vi "Check RPM.vi"(10 "Motor Input":dbl, 11 "RPM":dbl) -> (3 "RPM Drop":bool)   [LabVIEW 2013]
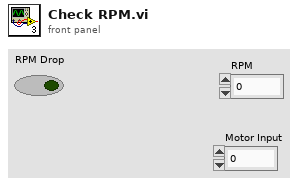
[diagram p1: front panel]
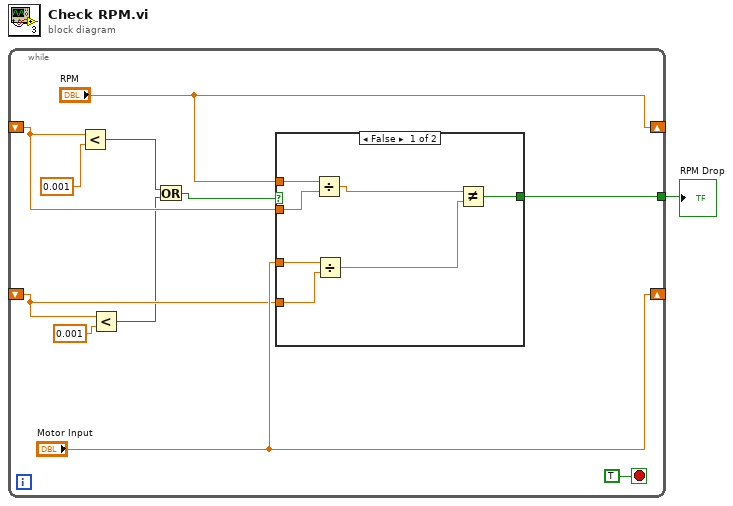
[diagram p0: block diagram]
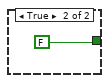
[diagram p2: hidden frame]
diagram:
  n1 = while {
    shift-right: ["RPM"] -> _
    shift-left: _ -> [w5]
    shift-right: ["Motor Input"] -> _
    shift-left: _ -> [w7]
    tunnel: [w9] -> w1
    stop <- TRUE stop-if-true
    n2 = Less?(x=w5, y=0.001) -> (x < y?=w4:bool)
    n3 = Less?(x=w7, y=0.001) -> (x < y?=w3:bool)
    n4 = Or(x=w4, y=w3) -> (x .or. y?=w2:bool)
    n5 = case shown="False" w2 {
      tunnel: [w19 FALSE] -> w9
      tunnel: "Motor Input" -> [w18 _]
      tunnel: w7 -> [w17 _]
      tunnel: "RPM" -> [w16 _]
      tunnel: w5 -> [w15 _]
      frame False {
        n6 = Divide(x=w16, y=w15) -> (x/y=w13:dbl)
        n7 = Divide(x=w18, y=w17) -> (x/y=w14:dbl)
        n8 = Not Equal?(x=w13, y=w14) -> (x != y?=w19:bool)
      }
      frame True {
      }
    }
  }
  "RPM Drop" <- w1
